vi "_Save RT Table.vi"(4 "error in (no error)":errorcluster, 6 "Table":dbl[][](array[numeric]), 7 "key":string) -> (0 "error out":errorcluster)   [LabVIEW 2012]
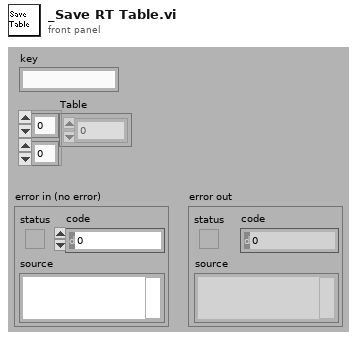
[diagram p1: front panel]
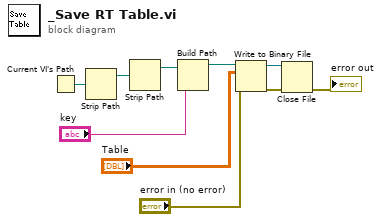
[diagram p0: block diagram]
diagram:
  n1 = Current VI's Path() -> (path=w8:path)
  n2 = Strip Path(path=w8) -> (stripped path=w9:path)  [unwired: 1 out]
  n3 = Strip Path(path=w9) -> (stripped path=w10:path)  [unwired: 1 out]
  n4 = Build Path(base path=w10, name or relative path="key") -> (appended path=w6:path)
  n5 = Write to Binary File(file (use dialog)=w6, data="Table", error in="error in (no error)") -> (refnum out=w3:refnum<file>, error out=w4:errorcluster)  [unwired: 4 out]
  n6 = Close File(refnum=w3, error in=w4) -> (error out=→"error out":errorcluster)  [unwired: 1 out]
